vi "Check Prompt Q.vi"(8 "error in (no error)":errorcluster, 11 "LoggingControl in":refnum<class "LoggingControl.lvclass">) -> (0 "error out":errorcluster, 3 "LoggingControl out":refnum<class "LoggingControl.lvclass">)   [LabVIEW 2020, in "VolatusGUIElements.lvlib" / "LoggingControl.lvclass"]
uses:
  LoggingControl.lvclass
  LoggingControl.lvclass/LoggingControl.ctl
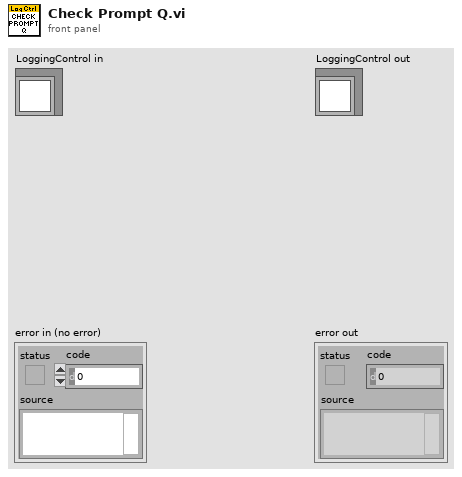
[diagram p1: front panel]
types:
  T1 = typedef "VolatusGUIElements.lvlib/LoggingControl.lvclass/Prompt Result.ctl" = cluster{"Action":T2, "Series":string, "Timestamp":string}
  T2 = typedef "VolatusGUIElements.lvlib/LoggingControl.lvclass/Prompt Action.ctl" = enum16{"Cancelled", "Started"}
  T3 = enum8{"Enabled", "Disabled", "Disabled and Grayed Out"}
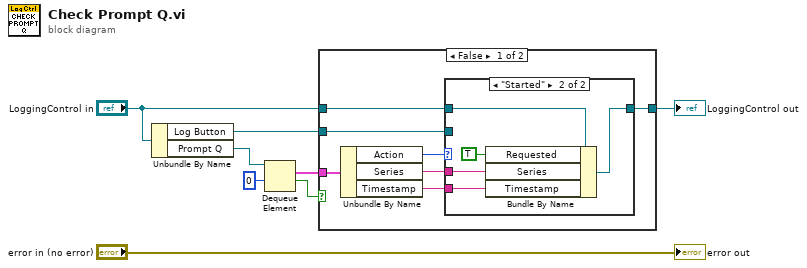
[diagram p0: block diagram]
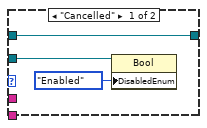
[diagram p2: hidden frame]
diagram:
  n1 = Unbundle By Name("LoggingControl in") -> ("Log Button"=w1:refnum<vi>, "Prompt Q"=w7:refnum<queue>)
  n2 = Dequeue Element(queue=w7, timeout in ms (-1)=0) -> (element=w3:T1, timed out?=w4:bool)  [unwired: 1 in, 2 out]
  n3 = case shown="False" w4 {
    tunnel: "LoggingControl in" -> [w14 w24]
    tunnel: w3 -> [w15 _]
    tunnel: [w10 w24] -> w2
    tunnel: w1 -> [w9 _]
    frame False {
      n4 = Unbundle By Name(w15) -> ("Action"=w13:T2, "Series"=w12:string, "Timestamp"=w11:string)
      n5 = case shown="\"Started\"" w13 {
        tunnel: w14 -> [w18 w23]
        tunnel: w12 -> [_ w22]
        tunnel: w11 -> [_ w20]
        tunnel: [w18 w19] -> w10
        tunnel: w9 -> [w17 _]
        frame "Cancelled" {
          n6 = property class="Bool"(reference=w17, "DisabledEnum"=T3."Enabled" ("Disabled")) -> ()  [unwired: 1 in, 2 out]
        }
        frame "Started" {
          n7 = Bundle By Name(cluster=w23, "Requested"=TRUE ("State.Requested"), "Series"=w22, "Timestamp"=w20) -> (w19:refnum<class "LoggingControl.lvclass">)
        }
      }
    }
    frame True {
    }
  }
  "LoggingControl out" <- w2
  "error out" <- "error in (no error)"
